vi "Case (Error IO)__ogtk.vi"() -> ()   [LabVIEW 2011]
doc: "Do not call this VI directly. This is a VI intended for\"merging\" into another VI, a case structure with \"error in\" and \"error out\" clusters."
panel:
  out "error out":errorcluster
  in  "error in (no error)":errorcluster
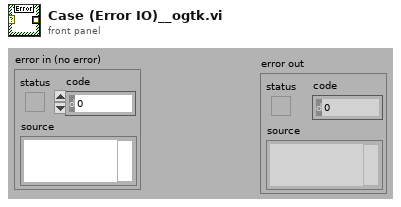
[diagram p1: front panel]
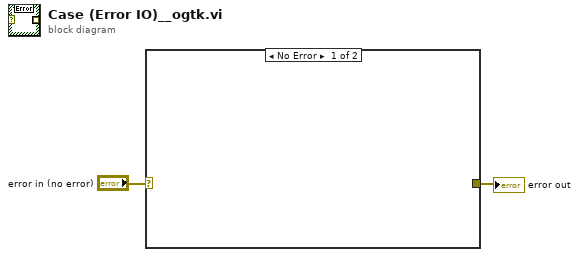
[diagram p0: block diagram]
diagram:
  n1 = case shown="No Error" "error in (no error)" {
    selector: "error in (no error)" -> [_ w3]
    tunnel: [_ w3] -> w1
    frame No Error {
    }
    frame Error {
    }
  }
  "error out" <- w1
